vi "QVA_ObtainQueue.vi"(1 "Name":string, 3 "InitValue":variant, 5 "ErrorIn":errorcluster) -> (14 "QueueOut":refnum<queue>, 17 "CreatedNew":bool, 19 "ErrorOut":errorcluster)   [LabVIEW 2016]
doc: "Erzeugt einen Variant Single Element Queue oder gibt die Referenz zurück, falls der Queue mit diesem Namen bereits existiert\n\nsige / 3.12.13"
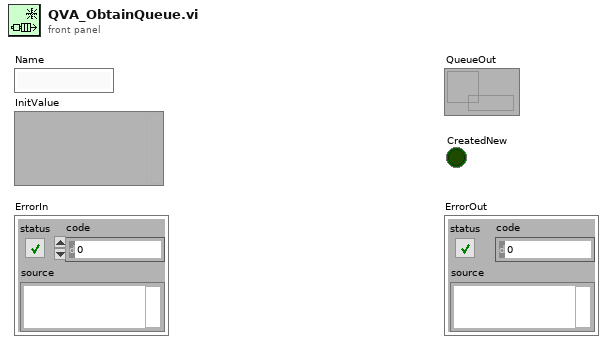
[diagram p1: front panel]
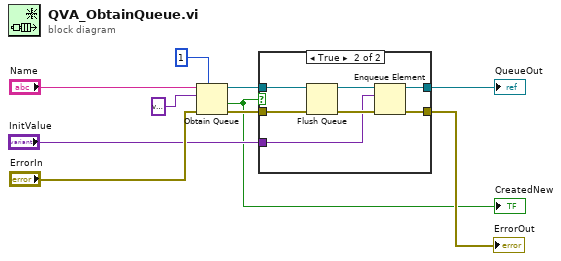
[diagram p0: block diagram]
diagram:
  n1 = Obtain Queue(max queue size (-1, unlimited)=1, name (unnamed)="Name", element data type=variant, error in (no error)="ErrorIn") -> (queue out=w6:refnum<queue>, created new?=w1:bool, error out=w5:errorcluster)  [unwired: 1 in]
  "CreatedNew" <- w1
  n2 = case shown="True" w1 {
    tunnel: w6 -> [w12 w19]
    tunnel: w5 -> [w11 w18]
    tunnel: "InitValue" -> [_ w15]
    tunnel: [w12 w14] -> w3
    tunnel: [w11 w13] -> w2
    frame False {
    }
    frame True {
      n3 = Flush Queue(queue=w19, error in (no error)=w18) -> (queue out=w17:refnum<queue>, error out=w16:errorcluster)  [unwired: 1 out]
      n4 = Enqueue Element(queue=w17, element=w15, error in (no error)=w16) -> (queue out=w14:refnum<queue>, error out=w13:errorcluster)  [unwired: 1 in, 1 out]
    }
  }
  "QueueOut" <- w3
  "ErrorOut" <- w2
